vi "LogBinaryArray.vi"(6 "Prepend Time?":bool, 8 "Array":dbl[](array[numeric]), 10 "Name":string, 11 "Path":path) -> ()   [LabVIEW 2012]
uses:
  <vilib>/addons/h5labview2/file/H5Fmode.ctl
  <vilib>/addons/h5labview2/file/H5F.lvlib
  <vilib>/addons/h5labview2/dataset/H5D.lvlib
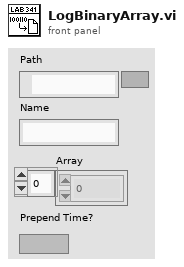
[diagram p1: front panel]
types:
  T1 = typedef "H5F.lvlib/H5Fmode.ctl" = enum16{"read-only", "read-write", "overwrite", "create new", "open or create"}
  T2 = typedef "hid_t.ctl" = i64
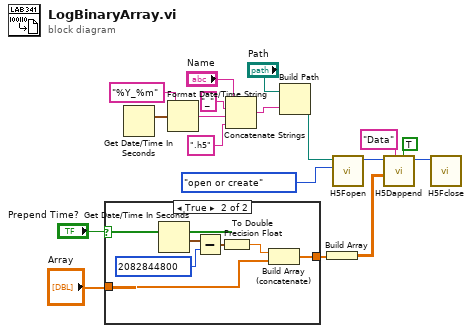
[diagram p0: block diagram]
diagram:
  n1 = case shown="True" "Prepend Time?" {
    tunnel: "Array" -> [w19 w25]
    tunnel: [w19 w20] -> w1
    frame False {
    }
    frame True {
      n2 = Get Date/Time In Seconds() -> (seconds since 1Jan1904=w24:timestamp)
      n3 = Subtract(x=w24, y=2082844800) -> (x-y=w23:timestamp)
      n4 = To Double Precision Float(number=w23) -> (double precision float=w21:dbl)
      n5 = Build Array (concatenate)(w21, w25) -> (w20:dbl[])
    }
  }
  n6 = Get Date/Time In Seconds() -> (seconds since 1Jan1904=w8:timestamp)
  n7 = Format Date/Time String(time format string (%c)="%Y_%m", seconds (now)=w8) -> (date/time string=w11:string)  [unwired: 1 in]
  n8 = Concatenate Strings("Name", "_", w11, ".h5" ("string")) -> (w10:string)
  n9 = Build Path(base path="Path", name or relative path=w10) -> (appended path=w4:path)
  n10 = Build Array(w1) -> (w18:dbl[][])
  n11 = call <vilib>:"H5Fopen.vi"("mode (read-only)"=H5Fmode."open or create", "path"=w4) -> ("ref out"=w16:T2)  [unwired: 8 in, 1 out]
  n12 = call <vilib>:"H5Dappend.vi"("create? (T)"=TRUE, "dataset name"="Data", "data"=w18, "ref in"=w16) -> ("ref out"=w15:T2)  [unwired: 4 in, 3 out]
  n13 = call <vilib>:"H5Fclose.vi"("ref"=w15) -> ()  [unwired: 10 in, 1 out]
